vi "getMatH.vi"(8 "error in (no error)":errorcluster, 10 "dofIdx":i32[](array[numeric]), 11 "OptCtrl in":refnum<class "OptCtrl.lvclass">) -> (0 "error out":errorcluster, 2 "Matrix H":dbl[][](array[numeric]), 3 "OptCtrl out":refnum<class "OptCtrl.lvclass">)   [LabVIEW 2016, in "OfcFunc.lvlib" / "OptCtrl.lvclass"]
doc: "Get the matrix H used in the control algorithm. It is noted that this matrix has considered the affection of penality on the authority of groups."
uses:
  OptCtrl.lvclass
  OptCtrl.lvclass/OptCtrl.ctl
  <vilib>/Analysis/7linalg.llb/Create Special Real Matrix.vi
  <vilib>/Analysis/Matrix/Numeric/Conversions/Matrix To Array - RM.vi
  MatOper/getSubArray2D.vi
  <vilib>/Analysis/NI_AALPro.lvlib
  <vilib>/Analysis/Matrix/NI_Matrix.lvlib
  MatOper/MatOper.lvclass
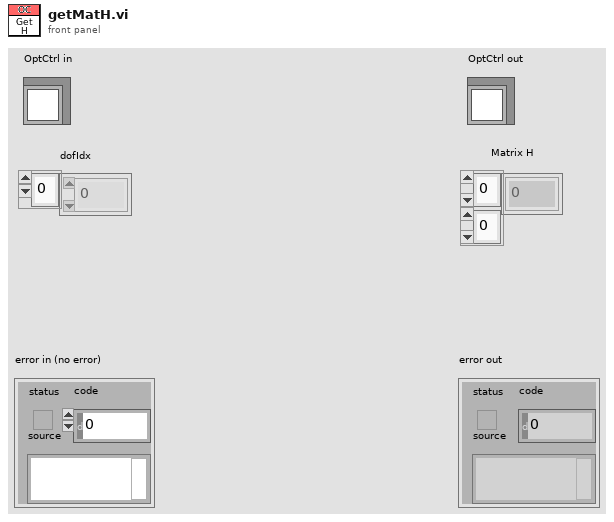
[diagram p1: front panel]
types:
  T1 = typedef "NI_Matrix.lvlib/RealMatrix.ctl" = dbl[][]
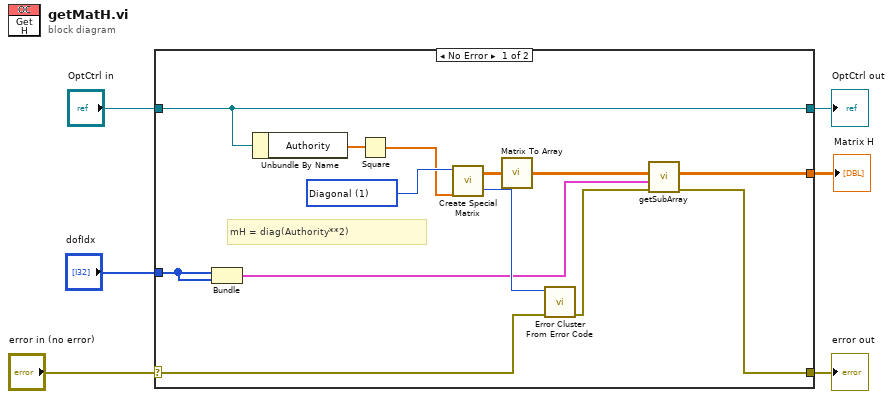
[diagram p0: block diagram]
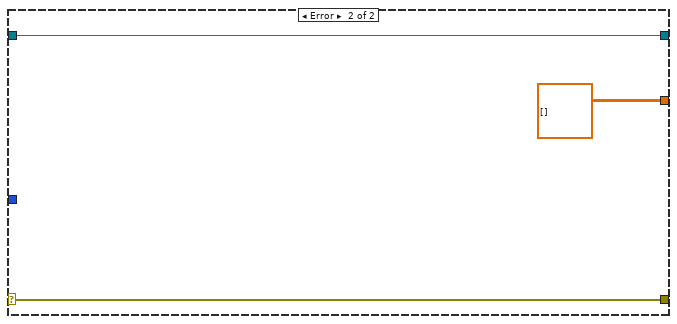
[diagram p2: hidden frame]
diagram:
  n1 = case shown="No Error" "error in (no error)" {
    selector: "error in (no error)" -> [w13 w22]
    tunnel: [w10 w22] -> w5
    tunnel: [w19 w21] -> w4
    tunnel: "OptCtrl in" -> [w19 w21]
    tunnel: [w7 dbl[][] [] ("Real 2D Array")] -> w3
    tunnel: "dofIdx" -> [w9 _]
    frame No Error {
      w17 = 1 items=["Identity", "Diagonal", "Toeplitz", "Vandermonde", "Companion", "Hankel", "Hadamard", "Wilkinson", "Hilbert", "Inverse Hilbert", "Rosser", "Pascal"] ("matrix type")
      # "mH = diag(Authority**2)"
      n2 = Bundle("dofIdx"=w9, "dofIdx"=w9) -> (w8:cluster{"dofIdx":i32[], "dofIdx":i32[]})  [unwired: 1 in]
      n3 = Unbundle By Name(w19) -> ("Authority"=w18:dbl[])
      n4 = Square(x=w18) -> (x^2=w16:dbl[])
      n5 = call-poly <vilib>:"Create Special Matrix.vi"("matrix type"=w17, "Input Vector1"=w16) -> ("Special Matrix"=w15:T1, "error"=w14:i32)  [unwired: 3 in]
      n6 = call-poly <vilib>:"Matrix To Array.vi"("Real Matrix"=w15) -> ("Real 2D Array"=w12:dbl[][])
      n7 = call <vilib>:"Error Cluster From Error Code.vi"("error in (no error)"=w13, "error code (0)"=w14) -> ("error out"=w11:errorcluster)  [unwired: 7 in]
      n8 = call-poly "getSubArray.vi"("error in (no error)"=w11, "Index Array Cluster"=w8, "2D Array"=w12) -> ("error out"=w10:errorcluster, "Sub-Array"=w7:dbl[][])  [unwired: 6 in, 1 out]
    }
    frame Error {
    }
  }
  "error out" <- w5
  "OptCtrl out" <- w4
  "Matrix H" <- w3
